vi "set_params.vi"(8 "error in (no error)":errorcluster caption="entrée d'erreur (pas d'erreur)", 11 "SGDClassifier.lvclass 2":refnum<class "SGDClassifier.lvclass">) -> (0 "error out":errorcluster caption="sortie d'erreur", 3 "SGDClassifier.lvclass":refnum<class "SGDClassifier.lvclass">)   [LabVIEW 2020, in "SGDClassifier.lvclass"]
uses:
  SGDClassifier.lvclass
  SGDClassifier.lvclass/SGDClassifier.ctl
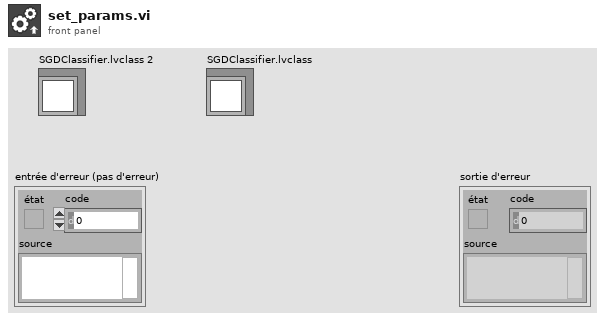
[diagram p1: front panel]
types:
  T1 = typedef "sgdclassifier_params.ctl" = cluster{"loss":string, "penalty":string, "alpha":dbl, "l1_ratio":dbl, "fit_intercept":bool, "max_iter":dbl, "tol":dbl, "shuffle":bool, "n_jobs":dbl, "random_state":dbl, "learning_rate":string, "eta0":dbl, "power_t":dbl, "early_stopping":bool, "validation_fraction":dbl, "n_iter_no_change":dbl, "class_weight":cluster{"class_weight_type":string, "class_weight_dict":string}, "warm_start":bool, "average":cluster{"average_type":string, "average_bool":bool, "average_int":dbl}}
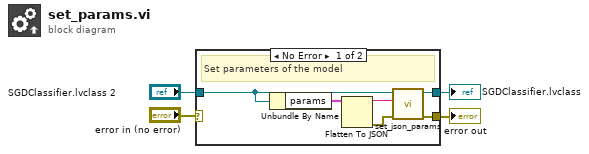
[diagram p0: block diagram]
diagram:
  n1 = case shown="No Error" "error in (no error)" {
    selector: "error in (no error)" -> [_ w12]
    tunnel: [w7 w12] -> w3
    tunnel: [w8 w11] -> w1
    tunnel: "SGDClassifier.lvclass 2" -> [w5 w11]
    frame No Error {
      # "Set parameters of the model"
      n2 = Unbundle By Name(w5) -> ("params"=w10:T1)
      n3 = Flatten To JSON(anything=w10) -> (JSON string=w9:string, 11:w6:errorcluster)  [unwired: 2 in]
      n4 = call-dynamic "set_json_params.vi"("error in (no error)"=w6, "params"=w9, "Model en entrée"=w5) -> ("error out"=w7:errorcluster, "Model en sortie"=w8:refnum<class "SGDClassifier.lvclass">)  [unwired: 7 in]
    }
    frame Error {
    }
  }
  "error out" <- w3
  "SGDClassifier.lvclass" <- w1
